vi "GetVIText.vi"(8 "error in (no error)":errorcluster, 10 "Control Name (Blank = All controls in VI)":string, 11 "VI":refnum<vi>) -> (0 "error out":errorcluster, 1 "Font Name":string, 2 "Control Text":string[](array[string]), 3 "Control Keys":string[](array[string]))   [LabVIEW 2017]
uses:
  <vilib>/Utility/traverseref.llb/TRef TravTarget.ctl
  <vilib>/Utility/traverseref.llb/VI Scripting - Traverse.lvlib
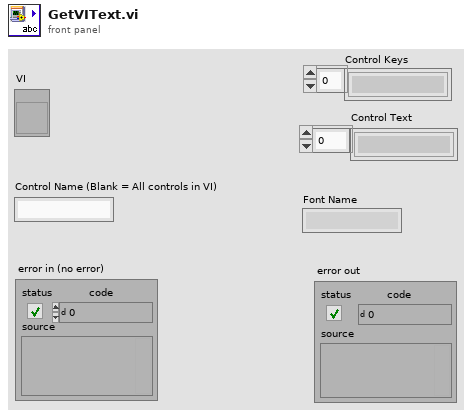
[diagram p1: front panel]
types:
  T1 = typedef "TRef TravTarget.ctl" = enum16{"FP", "BD", "Other"}
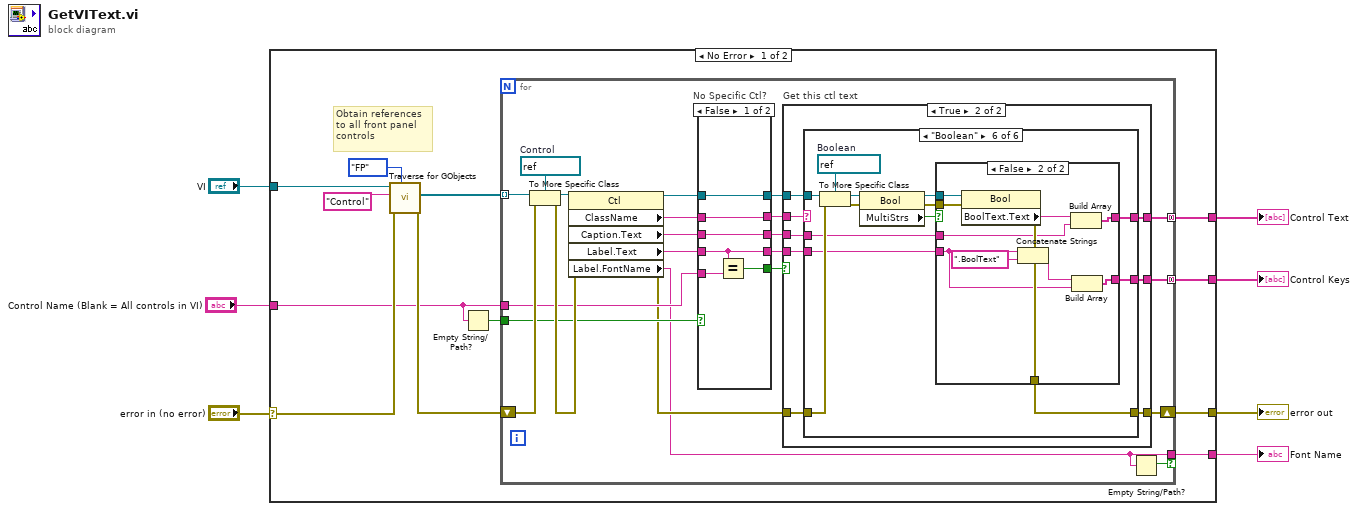
[diagram p0: block diagram]
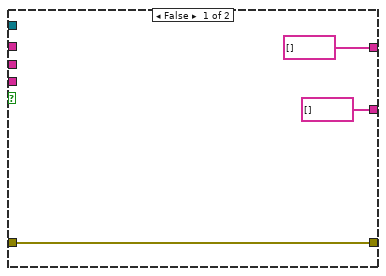
[diagram p2: hidden frame]
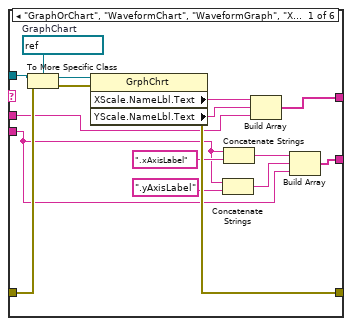
[diagram p3: hidden frame]
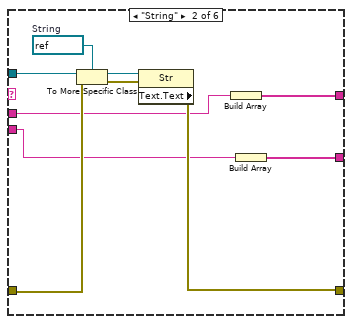
[diagram p4: hidden frame]
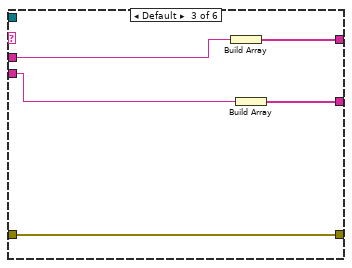
[diagram p5: hidden frame]
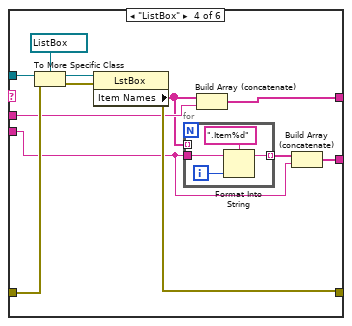
[diagram p6: hidden frame]
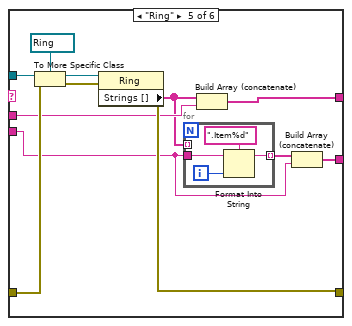
[diagram p7: hidden frame]
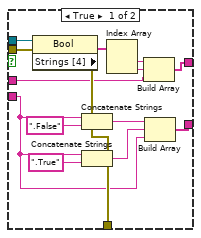
[diagram p8: hidden frame]
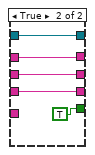
[diagram p9: hidden frame]
diagram:
  n1 = case shown="No Error" "error in (no error)" {
    selector: "error in (no error)" -> [w15 w164]
    tunnel: "VI" -> [w17 _]
    tunnel: "Control Name (Blank = All controls in VI)" -> [w11 _]
    tunnel: [w13 w164] -> w4
    tunnel: [w10 _] -> w3
    tunnel: [w9 _] -> w2
    tunnel: [w8 _] -> w1
    frame No Error {
      # "Obtain references to all front panel controls"
      n2 = call <vilib>:"Traverse for GObjects.vi"("Traverse Target"=TRef_TravTarget."FP", "error in (no error)"=w15, "Class Name"="Control", "VI Refnum"=w17) -> ("error out"=w14:errorcluster, "References"=w16:refnum<vi>[])  [unwired: 4 in, 2 out]
      n3 = Empty String/Path?(string/path=w11) -> (empty?=w12:bool)
      n4 = for {
        tunnel: w16 -> [w41] mode=indexing
        shift-right: [w30] -> w13
        shift-left: w14 -> [w38]
        tunnel: w11 -> [w36]
        tunnel: w12 -> [w34]
        tunnel: [w23] -> w10 mode=concatenating
        tunnel: [w22] -> w9 mode=concatenating
        tunnel: [w21] -> w8 if=w20
        w39 = refnum<vi> refnum  # Control
        n5 = To More Specific Class(target class=w39, reference=w41, error in=w38) -> (specific class reference=w40:refnum<vi>, error out=w37:errorcluster)
        n6 = property class="Ctl"(reference=w40, error in=w37) -> (reference out=w24:refnum<vi>, error out=w31:errorcluster, "ClassName"=w33:string, "Caption.Text"=w32:string, "Label.Text"=w35:string, "Label.FontName"=w21:string)
        n7 = case "No Specific Ctl?" shown="False" w34 {
          tunnel: w36 -> [w158 _]
          tunnel: w35 -> [w156 w160]
          tunnel: w33 -> [w154 w163]
          tunnel: w32 -> [w155 w161]
          tunnel: [w157 TRUE] -> w29
          tunnel: [w154 w163] -> w26
          tunnel: [w155 w161] -> w28
          tunnel: [w156 w160] -> w27
          tunnel: [w153 w159] -> w25
          tunnel: w24 -> [w153 w159]
          frame False {
            n8 = Equal?(x=w156, y=w158) -> (x = y?=w157:bool)
          }
          frame True {
          }
        }
        n9 = case "Get this ctl text" shown="True" w29 {
          tunnel: w31 -> [w44 w50]
          tunnel: [w44 w49] -> w30
          tunnel: w28 -> [_ w47]
          tunnel: w27 -> [_ w48]
          tunnel: w26 -> [_ w52]
          tunnel: w25 -> [_ w51]
          tunnel: [string[] [] w46] -> w23
          tunnel: [string[] [] w45] -> w22
          frame False {
          }
          frame True {
            n10 = case shown="\"Boolean\"" w52 {
              tunnel: w51 -> [w65 w75 _ w92 w108 w127]
              tunnel: w50 -> [w64 w74 w83 w91 w107 w126]
              tunnel: [w63 w73 w83 w90 w106 w125] -> w49
              tunnel: [w62 w72 w82 w89 w105 w124] -> w46
              tunnel: w48 -> [w54 w70 w80 w85 w101 w122]
              tunnel: w47 -> [w61 w71 w81 w88 w104 w123]
              tunnel: [w53 w69 w79 w84 w100 w121] -> w45
              frame "GraphOrChart", "WaveformChart", "WaveformGraph", "XYGraph" {
                w67 = refnum<vi> refnum  # GraphChart
                n11 = To More Specific Class(target class=w67, reference=w65, error in=w64) -> (specific class reference=w68:refnum<vi>, error out=w66:errorcluster)
                n12 = property class="GrphChrt"(reference=w68, error in=w66) -> (error out=w63:errorcluster, "XScale.NameLbl.Text"=w58:string, "YScale.NameLbl.Text"=w57:string)  [unwired: 1 out]
                n13 = Concatenate Strings(w54, ".yAxisLabel" ("string")) -> (w55:string)
                n14 = Concatenate Strings(w54, ".xAxisLabel" ("string")) -> (w56:string)
                n15 = Build Array(w58, w57, w61) -> (w62:string[])
                n16 = Build Array(w56, w55, w54) -> (w53:string[])
              }
              frame "String" {
                w78 = refnum<vi> refnum  # String
                n17 = To More Specific Class(target class=w78, reference=w75, error in=w74) -> (specific class reference=w77:refnum<vi>, error out=w76:errorcluster)
                n18 = property class="Str" props=["Text", "Text"](reference=w77, error in=w76) -> (error out=w73:errorcluster)  [unwired: 2 out]
                n19 = Build Array(w71) -> (w72:string[])
                n20 = Build Array(w70) -> (w69:string[])
              }
              frame Default {
                n21 = Build Array(w81) -> (w82:string[])
                n22 = Build Array(w80) -> (w79:string[])
              }
              frame "ListBox" {
                n23 = To More Specific Class(target class=refnum<vi> refnum ("reference out"), reference=w92, error in=w91) -> (specific class reference=w95:refnum<vi>, error out=w94:errorcluster)
                n24 = property class="LstBox"(reference=w95, error in=w94) -> (error out=w90:errorcluster, "Item Names"=w87:string[])  [unwired: 1 out]
                n25 = for {
                  tunnel: w85 -> [w99]
                  tunnel: w87 -> [_] mode=indexing
                  tunnel: [w96] -> w86 mode=indexing
                  i -> [w97]
                  n26 = Format Into String(format string=".Item%d", initial string=w99, w97) -> (resulting string=w96:string)  [unwired: 1 in, 1 out]
                }
                n27 = Build Array (concatenate)(w87, w88) -> (w89:string[])
                n28 = Build Array (concatenate)(w86, w85) -> (w84:string[])
              }
              frame "Ring" {
                n29 = To More Specific Class(target class=refnum<vi> refnum ("reference out"), reference=w108, error in=w107) -> (specific class reference=w111:refnum<vi>, error out=w110:errorcluster)
                n30 = property class="Ring"(reference=w111, error in=w110) -> (error out=w106:errorcluster, "Strings []"=w103:string[])  [unwired: 1 out]
                n31 = for {
                  tunnel: w101 -> [w115]
                  tunnel: w103 -> [_] mode=indexing
                  tunnel: [w112] -> w102 mode=indexing
                  i -> [w113]
                  n32 = Format Into String(format string=".Item%d", initial string=w115, w113) -> (resulting string=w112:string)  [unwired: 1 in, 1 out]
                }
                n33 = Build Array (concatenate)(w103, w104) -> (w105:string[])
                n34 = Build Array (concatenate)(w102, w101) -> (w100:string[])
              }
              frame "Boolean" {
                w128 = refnum<vi> refnum  # Boolean
                n35 = To More Specific Class(target class=w128, reference=w127, error in=w126) -> (specific class reference=w120:refnum<vi>, error out=w118:errorcluster)
                n36 = property class="Bool"(reference=w120, error in=w118) -> (reference out=w119:refnum<vi>, error out=w117:errorcluster, "MultiStrs"=w116:bool)
                n37 = case shown="False" w116 {
                  tunnel: [w142 w147] -> w125
                  tunnel: [w140 w151] -> w124
                  tunnel: w123 -> [w129 w143]
                  tunnel: w122 -> [w135 w144]
                  tunnel: [w134 w150] -> w121
                  tunnel: w119 -> [w133 w149]
                  tunnel: w117 -> [w132 w148]
                  frame True {
                    n38 = property class="Bool"(reference=w133, error in=w132) -> (error out=w142:errorcluster, "Strings [4]"=w141:string[])  [unwired: 1 out]
                    n39 = Concatenate Strings(w135, ".False" ("string")) -> (w138:string)
                    n40 = Concatenate Strings(w135, ".True" ("string")) -> (w136:string)
                    n41 = Index Array(array=w141) -> (element #1=w131:string, element #2=w130:string)  [unwired: 2 in]
                    n42 = Build Array(w131, w130, w129) -> (w140:string[])
                    n43 = Build Array(w138, w136, w135) -> (w134:string[])
                  }
                  frame False {
                    n44 = property class="Bool"(reference=w149, error in=w148) -> (error out=w147:errorcluster, "BoolText.Text"=w152:string)  [unwired: 1 out]
                    n45 = Concatenate Strings(w144, ".BoolText" ("string")) -> (w146:string)
                    n46 = Build Array(w152, w143) -> (w151:string[])
                    n47 = Build Array(w146, w144) -> (w150:string[])
                  }
                }
              }
            }
          }
        }
        n48 = Empty String/Path?(string/path=w21) -> (empty?=w20:bool)
      }
    }
    frame Error {
    }
  }
  "Control Text" <- w3
  "error out" <- w4
  "Control Keys" <- w2
  "Font Name" <- w1
